vi "XML_slow.vi"(1 "Slow Cluster":T1, 2 "Input String":string) -> (0 "Output String":string)   [LabVIEW 2012]
uses:
  Slow cluster control.ctl
panel:
  out "Descriptions":string[](array[string])
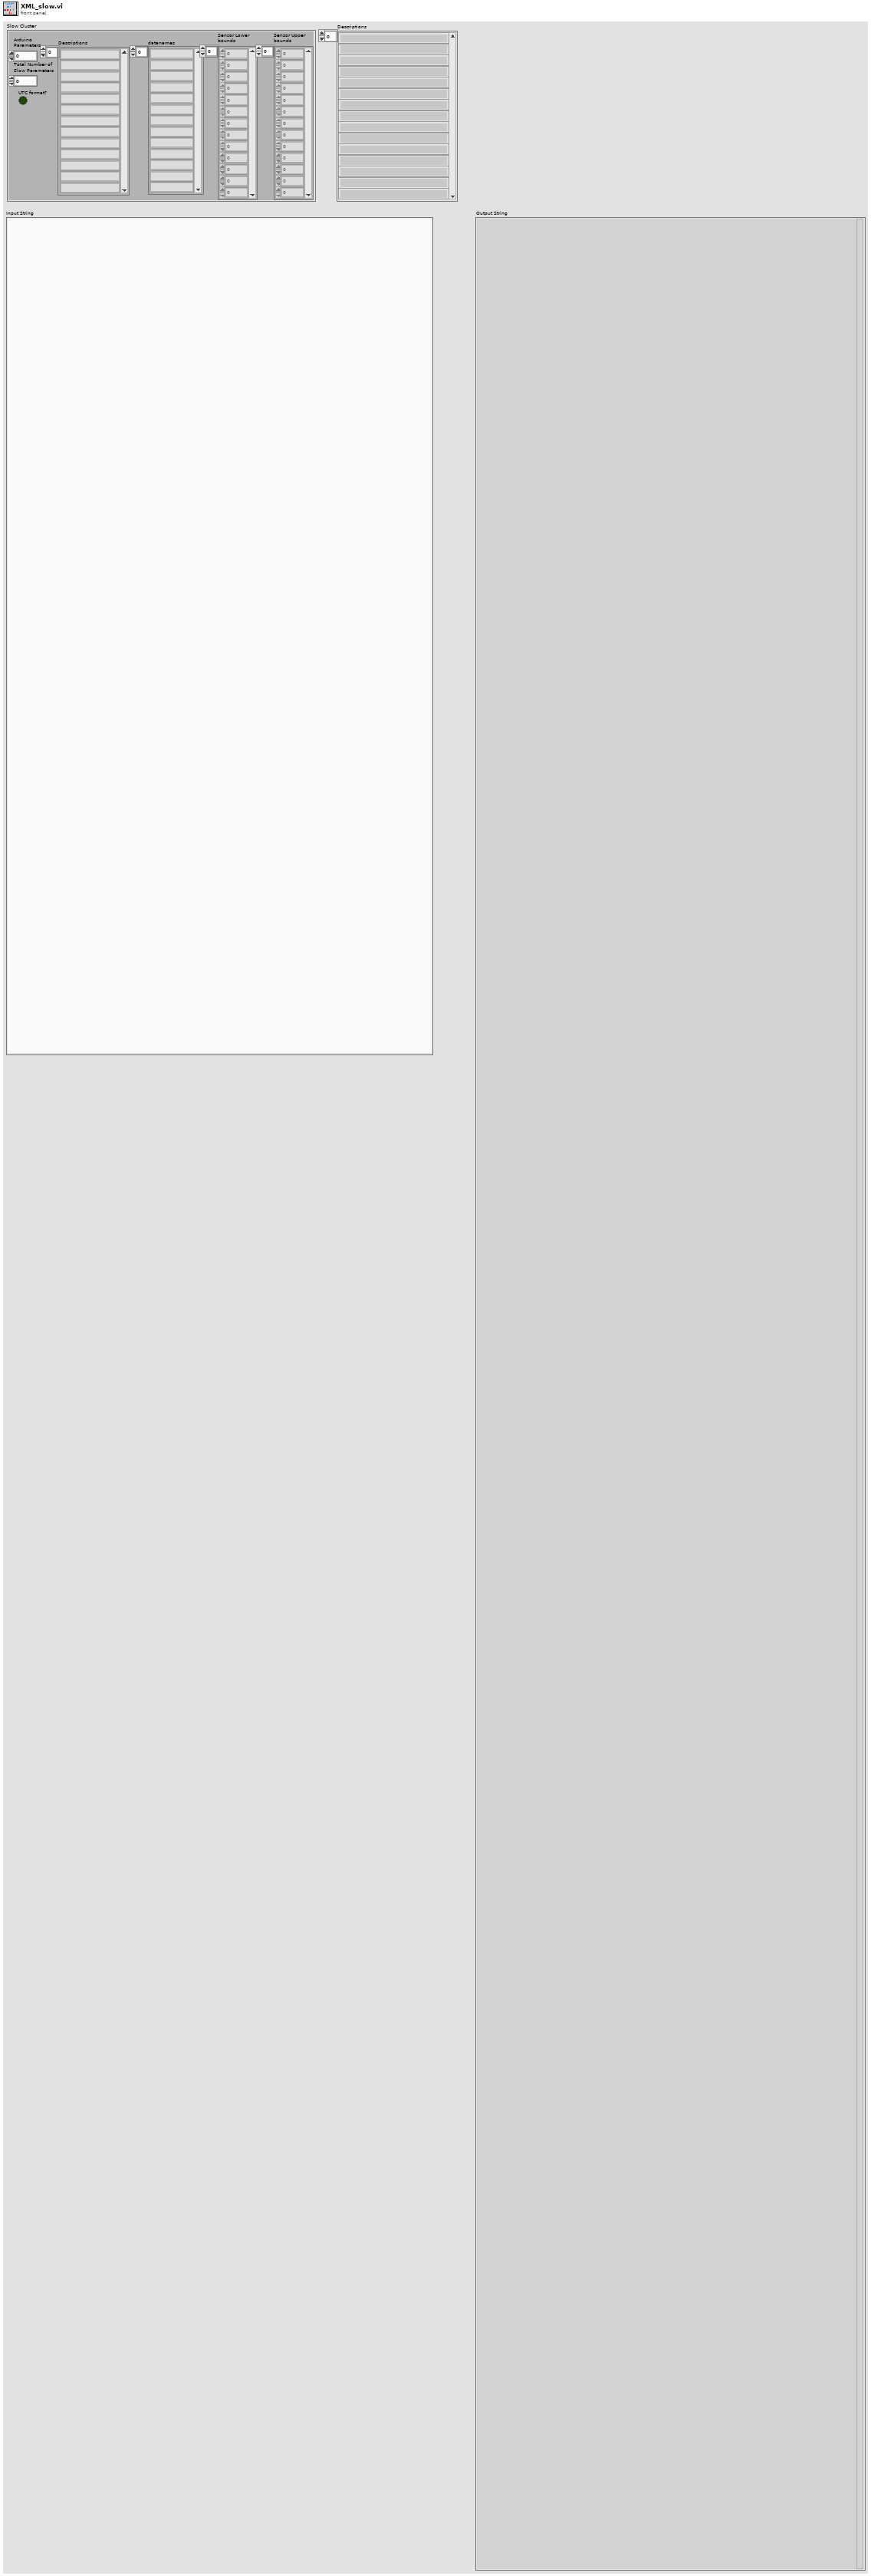
[diagram p1: front panel]
types:
  T1 = typedef "Slow cluster control.ctl" = cluster{"Arduino \nParameters":dbl, "Total Number of \nSlow Parameters":i32, "UTC format?":bool, "Sensor Upper \nbounds":i32[], "Sensor Lower \nbounds":i32[], "Descriptions":string[], "datanames":string[]}
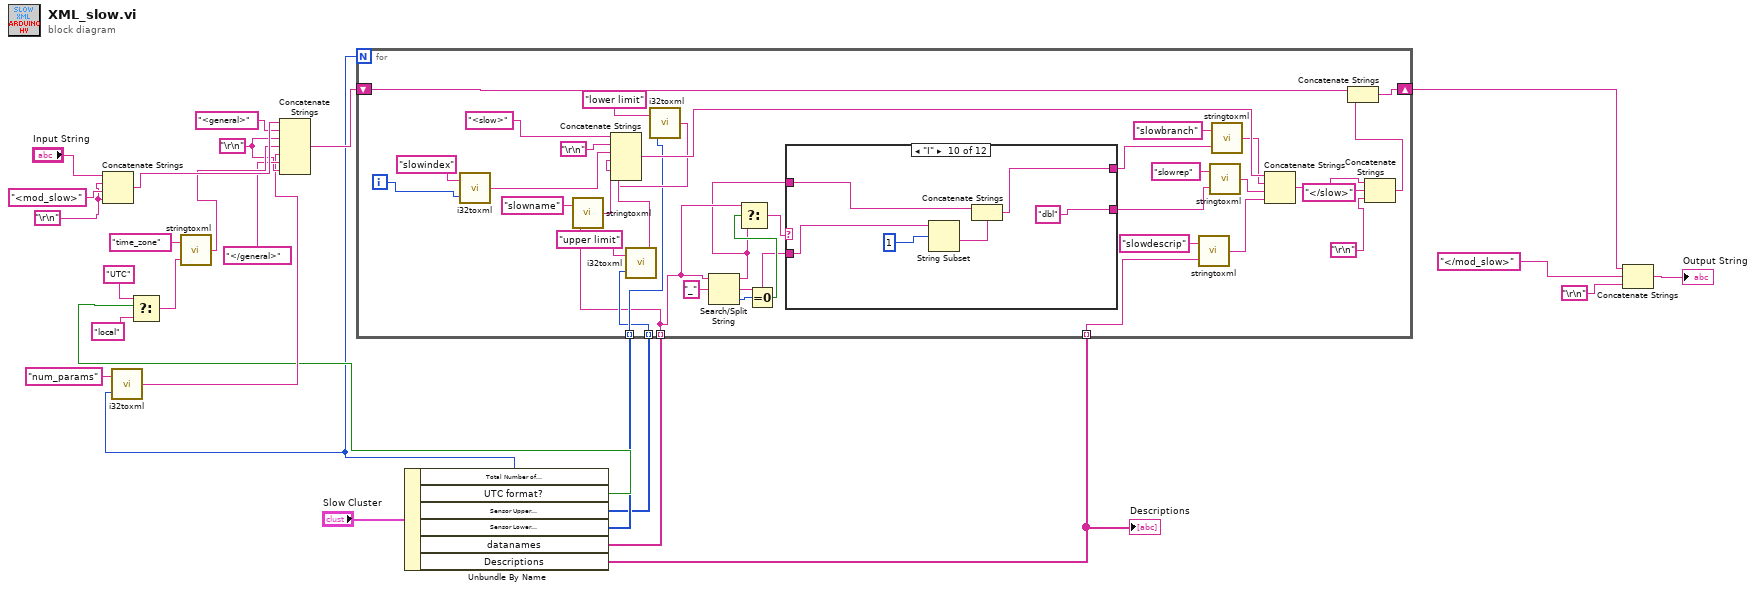
[diagram p0: block diagram]
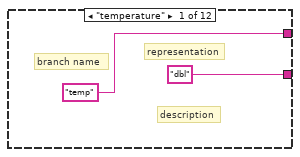
[diagram p2: hidden frame]
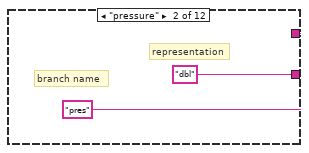
[diagram p3: hidden frame]
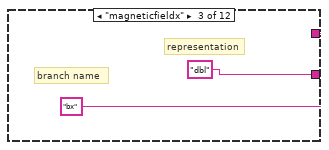
[diagram p4: hidden frame]
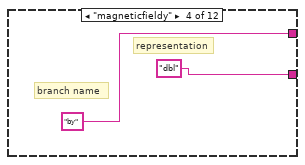
[diagram p5: hidden frame]
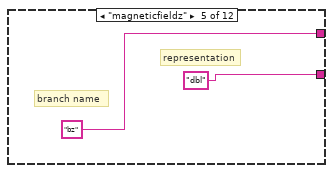
[diagram p6: hidden frame]
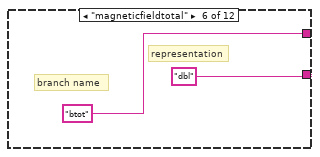
[diagram p7: hidden frame]
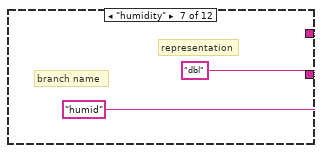
[diagram p8: hidden frame]
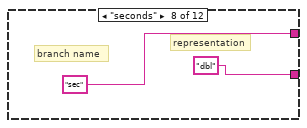
[diagram p9: hidden frame]
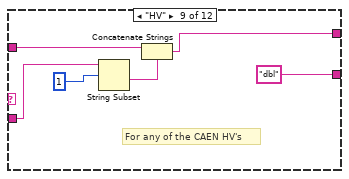
[diagram p10: hidden frame]
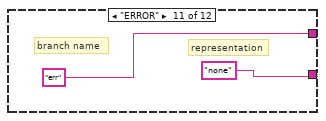
[diagram p11: hidden frame]
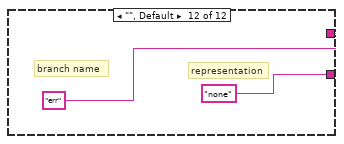
[diagram p12: hidden frame]
diagram:
  w16 = "\r\n"
  w1 = "\r\n"
  n1 = Concatenate Strings("Input String", w1, "<mod_slow>", w1) -> (w20:string)
  n2 = Unbundle By Name("Slow Cluster") -> ("Total Number of \nSlow Parameters"=w4:i32, "UTC format?"=w9:bool, "Sensor Upper \nbounds"=w7:i32[], "Sensor Lower \nbounds"=w8:i32[], "datanames"=w6:string[], "Descriptions"=w5:string[])
  "Descriptions" <- w5
  n3 = call "i32toxml.vi"("variable"=w4, "variable name"="num_params") -> ("xml string"=w13:string)
  n4 = Select(t="UTC" ("XML Tag"), s=w9, f="local") -> (s? t:f=w25:string)
  n5 = call "stringtoxml.vi"("String to write"=w25, "XML Tag"="time_zone") -> ("xml string"=w18:string)
  n6 = Concatenate Strings(w20, "<general>", w16, w18, w13, "</general>" ("string"), w16) -> (w12:string)
  n7 = for {
    N: w4 -> [_]
    shift-right: [w53] -> w10
    shift-left: w12 -> [w62]
    tunnel: w8 -> [w36] mode=indexing
    tunnel: w7 -> [w35] mode=indexing
    tunnel: w6 -> [w30] mode=indexing
    tunnel: w5 -> [w34] mode=indexing
    i -> [w37]
    n8 = call "i32toxml.vi"("variable"=w37, "variable name"="slowindex") -> ("xml string"=w43:string)
    n9 = call "stringtoxml.vi"("String to write"=w30, "XML Tag"="slowname") -> ("xml string"=w52:string)
    n10 = call "i32toxml.vi"("variable"=w35, "variable name"="upper limit") -> ("xml string"=w40:string)
    n11 = call "i32toxml.vi"("variable"=w36, "variable name"="lower limit") -> ("xml string"=w38:string)
    n12 = Concatenate Strings("<slow>" ("string"), "\r\n", w43, w52, w40, w38) -> (w50:string)
    n13 = Search/Split String(string=w30, search string/char (-)="_") -> (substring before match=w27:string, match + rest of string=w29:string, offset of match=w28:i32)  [unwired: 1 in]
    n14 = Equal To 0?(x=w28) -> (x = 0?=w32:bool)
    n15 = Select(t=w30, s=w32, f=w27) -> (s? t:f=w31:string)
    n16 = case shown="\"I\"" w31 {
      tunnel: ["dbl" ("XML Tag") "dbl" ("XML Tag") "dbl" ("XML Tag") "dbl" ("XML Tag") "dbl" ("XML Tag") "dbl" ("XML Tag") "dbl" ("XML Tag") "dbl" ("XML Tag") "dbl" ("XML Tag") "dbl" ("XML Tag") "none" ("XML Tag") "none" ("XML Tag")] -> w58
      tunnel: ["temp" "pres" "bx" "by" "bz" "btot" "humid" "sec" w81 w85 "err" "err"] -> w47
      tunnel: w29 -> [_ _ _ _ _ _ _ _ w83 w87 _ _]
      tunnel: w27 -> [_ _ _ _ _ _ _ _ w80 w88 _ _]
      frame "temperature" {
        # "branch name"
        # "description"
        # "representation"
      }
      frame "pressure" {
        # "branch name"
        # "representation"
      }
      frame "magneticfieldx" {
        # "branch name"
        # "representation"
      }
      frame "magneticfieldy" {
        # "branch name"
        # "representation"
      }
      frame "magneticfieldz" {
        # "branch name"
        # "representation"
      }
      frame "magneticfieldtotal" {
        # "branch name"
        # "representation"
      }
      frame "humidity" {
        # "branch name"
        # "representation"
      }
      frame "seconds" {
        # "branch name"
        # "representation"
      }
      frame "HV" {
        # "For any of the CAEN HV's"
        n17 = String Subset(string=w83, offset (0)=1) -> (substring=w82:string)  [unwired: 1 in]
        n18 = Concatenate Strings(w80, w82) -> (w81:string)
      }
      frame "I" {
        n19 = String Subset(string=w87, offset (0)=1) -> (substring=w90:string)  [unwired: 1 in]
        n20 = Concatenate Strings(w88, w90) -> (w85:string)
      }
      frame "ERROR" {
        # "branch name"
        # "representation"
      }
      frame "", Default {
        # "branch name"
        # "representation"
      }
    }
    n21 = call "stringtoxml.vi"("String to write"=w34, "XML Tag"="slowdescrip") -> ("xml string"=w56:string)
    n22 = call "stringtoxml.vi"("String to write"=w58, "XML Tag"="slowrep") -> ("xml string"=w57:string)
    n23 = call "stringtoxml.vi"("String to write"=w47, "XML Tag"="slowbranch") -> ("xml string"=w49:string)
    n24 = Concatenate Strings(w50, w49, w57, w56) -> (w51:string)
    n25 = Concatenate Strings(w51, "</slow>" ("string"), "\r\n") -> (w54:string)
    n26 = Concatenate Strings(w62, w54) -> (w53:string)
  }
  n27 = Concatenate Strings(w10, "</mod_slow>" ("string"), "\r\n") -> (→"Output String":string)
